vi "HTTP TCP No Timeout Error.vi"(4 "Restart Timeout?":bool, 6 "Timeout ms (-1)":i32=-1, 9 "error in (no error)":errorcluster) -> (0 "timeout expired?":bool, 1 "error out":errorcluster)   [LabVIEW 2011]
panel:
  out "timeout counter":u32
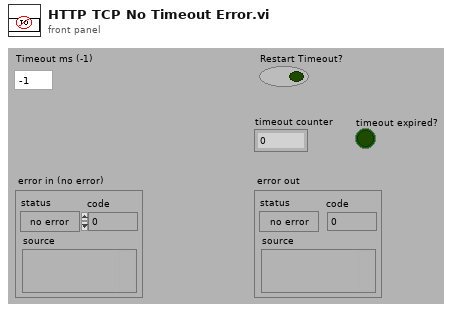
[diagram p1: front panel]
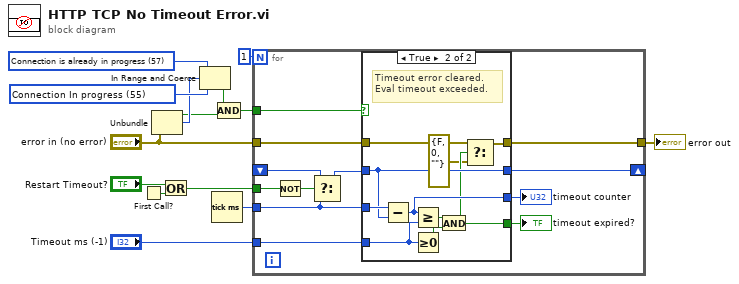
[diagram p0: block diagram]
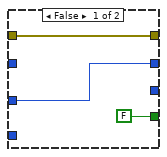
[diagram p2: hidden frame]
diagram:
  w1 = u16 57 items=["No Error", "Argument Error", "Memory Full", "Out of Zone", "End of File", "File Already Open", "Generic File IO Error", "File Not Found", "File Permission Error", "Disk Full", "Duplicate Path", "Too Many Files Open", "Not Enabled", "Resource File Not Found", "Cannot Add Resource", "Resource Not Found", "Image Not Found", "Image Memory Error", "Pen Does Not Exist", "Config Bad Type", "Config Token Not Found", "Config Parse Error", "Config Memory Error", "Bad External Code Format", "Bad External Code Offset", "External Code Not Present", "Null Window", "Destroy Window Mixup", "Null Menu", "Print Aborted", "Bad Print Record", "Print Driver Error", "Windows Error During Print", "Memory Error During Print", "Print Dialog Error", "Generic Print Error", "Invalid Device Refnum", "Device Not Found", "Device Parameter Error", "Device Unit Error", "Can't Open Device", "Device Call Aborted", "Generic Error", "Cancelled By User", "Object ID Too Low", "Object ID Too High", "Object Not In Heap", "Unknown Heap", "Bad DefProc ID", "DefProc Not In Table", "Message Out Of Range", "Null Method", "Unknown Message", "Manager Call Not Supported", "Bad address", "Connection In progress", "Connection timed out", "Connection is already in progress", "Network attribute not supported", "Network error", "Address in use", "System out of memory", "Connection aborted", "Connection refused", "Connection is not connected", "Connection is already connected", "Connection closed", "Initialize error (interapplication manager)", "Bad occurrence", "Wait on unbound occurrence handler", "Occurrence queue overflow", "Bad path", "Semaphore not signaled", "Unrecognized type (interapplication manager)"]
  w14 = u16 55 items=["No Error", "Argument Error", "Memory Full", "Out of Zone", "End of File", "File Already Open", "Generic File IO Error", "File Not Found", "File Permission Error", "Disk Full", "Duplicate Path", "Too Many Files Open", "Not Enabled", "Resource File Not Found", "Cannot Add Resource", "Resource Not Found", "Image Not Found", "Image Memory Error", "Pen Does Not Exist", "Config Bad Type", "Config Token Not Found", "Config Parse Error", "Config Memory Error", "Bad External Code Format", "Bad External Code Offset", "External Code Not Present", "Null Window", "Destroy Window Mixup", "Null Menu", "Print Aborted", "Bad Print Record", "Print Driver Error", "Windows Error During Print", "Memory Error During Print", "Print Dialog Error", "Generic Print Error", "Invalid Device Refnum", "Device Not Found", "Device Parameter Error", "Device Unit Error", "Can't Open Device", "Device Call Aborted", "Generic Error", "Cancelled By User", "Object ID Too Low", "Object ID Too High", "Object Not In Heap", "Unknown Heap", "Bad DefProc ID", "DefProc Not In Table", "Message Out Of Range", "Null Method", "Unknown Message", "Manager Call Not Supported", "Bad address", "Connection In progress", "Connection timed out", "Connection is already in progress", "Network attribute not supported", "Network error", "Address in use", "System out of memory", "Connection aborted", "Connection refused", "Connection is not connected", "Connection is already connected", "Connection closed", "Initialize error (interapplication manager)", "Bad occurrence", "Wait on unbound occurrence handler", "Occurrence queue overflow", "Bad path", "Semaphore not signaled", "Unrecognized type (interapplication manager)"]
  n1 = First Call?() -> (First Call?: T/F=w5:bool)
  n2 = Unbundle("error in (no error)") -> ("status"=w8:bool, "code"=w12:i32)  [unwired: 1 out]
  n3 = Or(x="Restart Timeout?", y=w5) -> (x .or. y?=w3:bool)
  n4 = In Range and Coerce(upper limit=w1, x=w12, lower limit=w14) -> (In Range?=w13:bool)  [unwired: 1 out]
  n5 = Tick Count (ms)() -> (millisecond timer value=w7:u32)
  n6 = Compound Arithmetic op=AND(w13, w8) -> (w9:bool)
  n7 = for {
    N: 1 -> [_]
    tunnel: [w26] -> w11
    tunnel: "error in (no error)" -> [w25]
    tunnel: w9 -> [w24]
    shift-right: [w17] -> _
    shift-left: _ -> [w23]
    tunnel: w7 -> [w21]
    tunnel: "Timeout ms (-1)" -> [w20]
    tunnel: w3 -> [w18]
    n8 = Not(x=w18) -> (.not. x?=w19:bool)
    n9 = Select(t=w23, s=w19, f=w21) -> (s? t:f=w22:u32)
    n10 = case shown="True" w24 {
      tunnel: w25 -> [w29 w32]
      tunnel: [w29 w30] -> w26
      tunnel: w22 -> [_ w38]
      tunnel: [w28 w38] -> w17
      tunnel: w21 -> [w28 w39]
      tunnel: w20 -> [_ w37]
      tunnel: [FALSE w33] -> w16
      tunnel: [_ w34] -> w15
      frame False {
      }
      frame True {
        # "Timeout error cleared. Eval timeout exceeded."
        n11 = Subtract(x=w39, y=w38) -> (x-y=w34:u32)
        n12 = Greater Or Equal?(x=w34, y=w37) -> (x >= y?=w35:bool)
        n13 = Greater Or Equal To 0?(x=w37) -> (x >= 0?=w36:bool)
        n14 = And(x=w35, y=w36) -> (x .and. y?=w33:bool)
        n15 = Select(t=w32, s=w33, f=errorcluster {"status"=FALSE, "code"=0, "source"=""}) -> (s? t:f=w30:errorcluster)
      }
    }
    "timeout expired?" <- w16
    "timeout counter" <- w15
  }
  "error out" <- w11
